vi "Database Structure.vi"(0 "InfluxDB in":refnum<class "Client.lvclass">, 5 "Database name":string, 11 "error in (no error)":errorcluster) -> (4 "InfluxDB out":refnum<class "Client.lvclass">, 8 "Field keys":refnum<class "Results.lvclass">, 10 "Tag keys":refnum<class "Results.lvclass">, 15 "error out":errorcluster)   [LabVIEW 2018, in "InfluxDB Client.lvlib" / "Client.lvclass"]
doc: "Creates a database."
uses:
  Client.lvclass
  Results/Results.lvclass
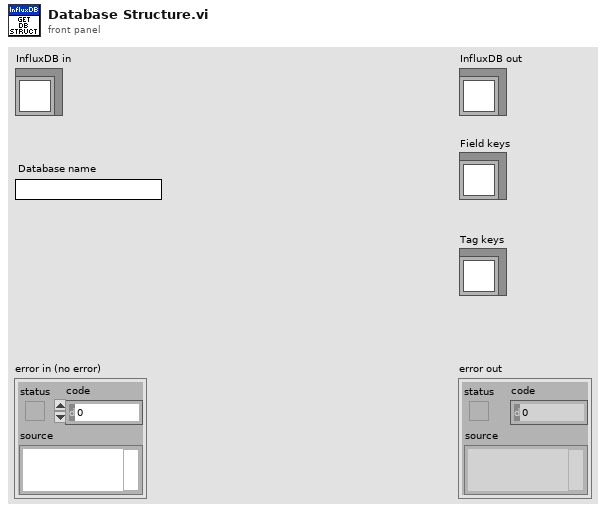
[diagram p1: front panel]
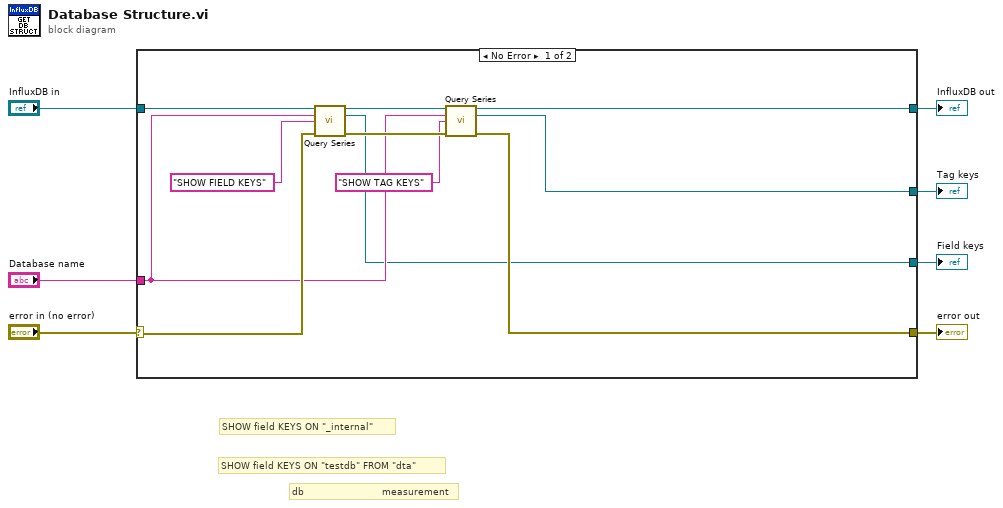
[diagram p0: block diagram]
diagram:
  # "db                          measurement"
  # "SHOW field KEYS ON \"testdb\" FROM \"dta\""
  # "SHOW field KEYS ON \"_internal\""
  n1 = case shown="No Error" "error in (no error)" {
    selector: "error in (no error)" -> [w17 w20]
    tunnel: [w12 w20] -> w6
    tunnel: [w11 w19] -> w4
    tunnel: "InfluxDB in" -> [w18 w19]
    tunnel: "Database name" -> [w10 _]
    tunnel: [w9 _] -> w2
    tunnel: [w8 _] -> w1
    frame No Error {
      n2 = call "Query Series.vi"("InfluxDB in"=w18, "Database name"=w10, "Measurement query"="SHOW FIELD KEYS", "error in (no error)"=w17) -> ("InfluxDB out"=w15:refnum<class "Client.lvclass">, "Results Out"=w8:refnum<class "Results.lvclass">, "error out"=w14:errorcluster)  [unwired: 9 in]
      n3 = call "Query Series.vi"("InfluxDB in"=w15, "Database name"=w10, "Measurement query"="SHOW TAG KEYS", "error in (no error)"=w14) -> ("InfluxDB out"=w11:refnum<class "Client.lvclass">, "Results Out"=w9:refnum<class "Results.lvclass">, "error out"=w12:errorcluster)  [unwired: 9 in]
    }
    frame Error {
    }
  }
  "error out" <- w6
  "InfluxDB out" <- w4
  "Tag keys" <- w2
  "Field keys" <- w1
